vi "Actor Core.vi"(8 "error in":errorcluster, 11 "Open File in":refnum<class "Open File.lvclass">) -> (0 "error out":errorcluster, 3 "Actor out":refnum<class "Actor.lvclass">)   [LabVIEW 2018, in "Open File Actor.lvlib" / "Open File.lvclass"]
doc: "(<B>Filename</B>: Actor Framework.lvlib:Actor.lvclass:Actor Core.vi)\n\nReceives messages to the actor, reacts to them, and initiates any error handling that may shut the actor down.\n\nDescendant classes may override this VI to append parallel tasks for the actor to complete while it handles messages. Overrides use the Call Parent Method node."
uses:
  Open File.lvclass
  C:/Program Files (x86)/National Instruments/LabVIEW 2018/vi.lib/ActorFramework/Actor/Actor.lvclass
  <vilib>/ActorFramework/Actor/Actor.lvclass
  <vilib>/ActorFramework/Actor/Actor.lvclass/Actor.ctl
  <vilib>/ActorFramework/Message Enqueuer/Message Enqueuer.lvclass/Message Enqueuer.ctl
  Open File.lvclass/Open File.ctl
  Open File Messages/File Data Msg/File Data Msg.lvclass/File Data Msg.ctl
  <vilib>/ActorFramework/Message Enqueuer/Init from Existing Queue.vi
  <vilib>/ActorFramework/Message Enqueuer/Enqueue.vi
  Open File Messages/File Data Msg/File Data Msg.lvclass
  C:/Program Files (x86)/National Instruments/LabVIEW 2018/vi.lib/ActorFramework/Message/Message.lvclass
  <vilib>/ActorFramework/Stop Msg/Stop Msg.lvclass
  <vilib>/ActorFramework/Message Priority Queue/Priority Enqueue.vi
  <vilib>/ActorFramework/Message Enqueuer/Message Enqueuer.lvclass
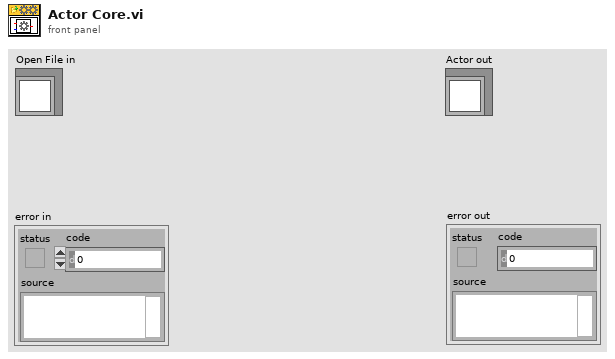
[diagram p1: front panel]
types:
  T1 = enum16{"open", "replace", "create", "open or create", "replace or create", "replace or create with confirmation"}
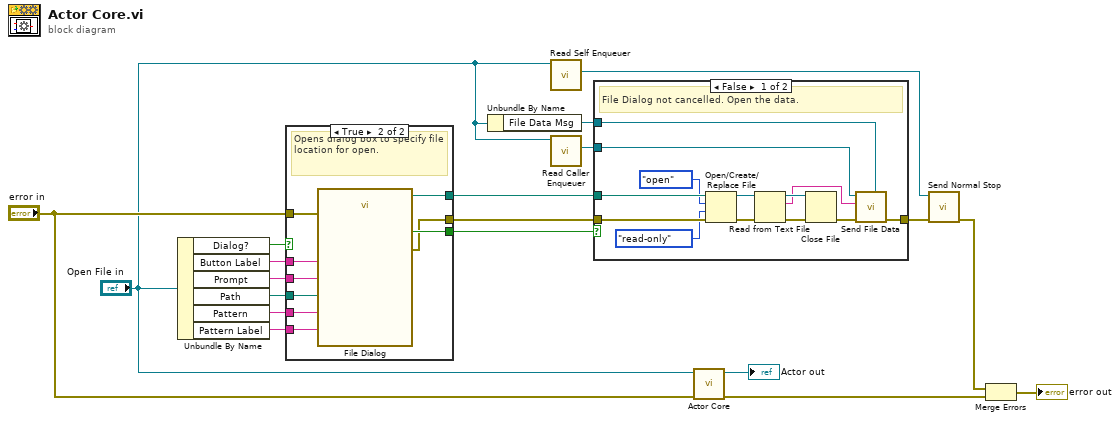
[diagram p0: block diagram]
diagram:
  n1 = Unbundle By Name("Open File in") -> ("Dialog?"=w17:bool, "Button Label"=w16:string, "Prompt"=w15:string, "Path"=w14:path, "Pattern"=w13:string, "Pattern Label"=w12:string)
  n2 = case shown="True" w17 {
    tunnel: w16 -> [_ w30]
    tunnel: w15 -> [_ w29]
    tunnel: w14 -> [w20 w28]
    tunnel: w13 -> [_ w27]
    tunnel: w12 -> [_ w26]
    tunnel: [_ w25] -> w10
    tunnel: [w20 w24] -> w9
    tunnel: "error in" -> [w21 w23]
    tunnel: [w21 w22] -> w8
    frame False {
      # "Passes the path through to save the file."
    }
    frame True {
      # "Opens dialog box to specify file location for open."
      n3 = call "File Dialog"("start path"=w28, "prompt"=w29, "button label"=w30, "error in"=w23, "pattern (all files)"=w27, "pattern label"=w26) -> ("selected path"=w24:path, "cancelled"=w25:bool, "error out"=w22:errorcluster)  [unwired: 6 in, 1 out]
    }
  }
  n4 = Unbundle By Name("Open File in") -> ("File Data Msg"=w7:refnum<class "File Data Msg.lvclass">)
  n5 = call <vilib>:"Read Self Enqueuer.vi"("Actor"="Open File in") -> ("Self Enqueuer"=w3:refnum<class "Message Enqueuer.lvclass">)  [unwired: 10 in]
  n6 = call <vilib>:"Read Caller Enqueuer.vi"("Actor"="Open File in") -> ("Caller Enqueuer"=w2:refnum<class "Message Enqueuer.lvclass">)  [unwired: 10 in]
  n7 = case shown="False" w10 {
    tunnel: w9 -> [w43 _]
    tunnel: w8 -> [w42 w44]
    tunnel: w7 -> [w32 _]
    tunnel: [w34 w44] -> w4
    tunnel: w2 -> [w33 _]
    frame False {
      # "File Dialog not cancelled. Open the data."
      n8 = Open/Create/Replace File(file path (use dialog)=w43, error in=w42, operation (0:open)=T1."open", access (0:read/write)=enum16{"read/write", "read-only", "write-only"}."read-only") -> (refnum out=w39:refnum<file>, error out=w38:errorcluster)  [unwired: 2 in, 1 out]
      n9 = Read from Text File(file (use dialog)=w39, error in=w38) -> (refnum out=w36:refnum<file>, text=w31:string, error out=w37:errorcluster)  [unwired: 2 in, 1 out]
      n10 = Close File(refnum=w36, error in=w37) -> (error out=w35:errorcluster)  [unwired: 1 out]
      n11 = call "Send File Data.vi"("Message Type"=w32, "error in (no error)"=w35, "Data"=w31, "Message Enqueuer"=w33) -> ("error out"=w34:errorcluster)  [unwired: 6 in, 1 out]
    }
    frame True {
      # "Do nothing if the File Dialog was cancelled."
    }
  }
  n12 = call-parent "Actor Core.vi"("error in"="error in", "Actor in"="Open File in") -> ("error out"=w19:errorcluster, "Actor out"=→"Actor out":refnum<class "Actor.lvclass">)  [unwired: 8 in]
  n13 = call <vilib>:"Send Normal Stop.vi"("error in (no error)"=w4, "Message Enqueuer"=w3) -> ("error out"=w5:errorcluster)  [unwired: 9 in]
  n14 = Merge Errors(w5, w19) -> (→"error out":errorcluster)
